vi "ToRepo.vi"(8 "error in":errorcluster, 9 "to repo cluster":T1, 10 "repository in":refnum<class "NISE_CEF_Repository.lvclass">, 11 "node in":refnum<class "Pages.lvclass">) -> (0 "error out":errorcluster, 2 "repository out":refnum<class "NISE_CEF_Repository.lvclass">, 3 "node out":refnum<class "Pages.lvclass">)   [LabVIEW 2015, in "Pages.lvclass"]
doc: "Transfers the information from the tree node into the repo. How it is stored in the repo depends on the Repo.Copyright 2015 National Instruments Corporation\n\nLicensed under the Apache License, Version 2.0 (the \"License\"); you may not use this file except in compliance with the License. You may obtain a copy of the License at http://www.apache.org/licenses/LICENSE-2.0\nUnless required by applicable law or agreed to in writing, software distributed under the License is distributed on an \"AS IS\" BASIS, WITHOUT WARRANTIES OR CONDITIONS OF ANY KIND, either express or implied. See the License for the specific language governing permissions and limitations under the License."
uses:
  Pages.lvclass
  <vilib>/NI/Configuration Framework/Repository/NISE_CEF_Repository.lvclass
  <vilib>/NI/Configuration Framework/Node/ToRepoCluster.ctl
  CustomDeviceRepo/CustomDeviceRepo.lvclass
  <vilib>/NI/Configuration Framework/Node/NISE_CEF_Node.lvclass/NISE_CEF_Node.ctl
  Page/Page.lvclass
  Custom Device Type Defs/Page Properties.ctl
  XML Controls/Path Cluster.ctl
  XML Controls/help.ctl
  Custom Device Type Defs/ActionVIs Properties.ctl
  Custom Device Type Defs/ButtonLists Properties.ctl
  XML Controls/Button Type.ctl
  XML Controls/Dependency three item small.ctl
  Custom Device Type Defs/RunTimeMenus Properties.ctl
  XML Controls/Execution Types.ctl
  Page/Page.lvclass/Page.ctl
  RunTimeObjects/RunTimeObjectsSection.lvclass
  RunTimeObjects/RunTimeObjectsSection.lvclass/RunTimeObjectsSection.ctl
  ActionVI/ActionVI.lvclass
  ActionVI/ActionVI.lvclass/ActionVI.ctl
  RunTimeButton/RunTimeButton.lvclass
  RunTimeButton/RunTimeButton.lvclass/RunTimeButton.ctl
  RunTimeMenuItem/RunTimeMenuItem.lvclass
  RunTimeMenuItem/RunTimeMenuItem.lvclass/RunTimeMenuItem.ctl
  CustomDeviceRepo/CustomDeviceRepo.lvclass/CustomDeviceRepo.ctl
  ActionVI/Read ActionVIType.vi
  ActionVI/Read Action VI Properties.vi
  RunTimeButton/Read Button Properties.vi
  RunTimeMenuItem/Read Run Time Menu Properties.vi
  RunTimeObjects/Read RunTimeObjectType.vi
  <vilib>/NI/Configuration Framework/Node/ReadChildren.vi
  Page/Read General Page Properties.vi
  CustomDeviceRepo/Write All Pages Properties.vi
  <vilib>/NI/Configuration Framework/Node/NISE_CEF_Node.lvclass
  Configuration Tool.lvlib
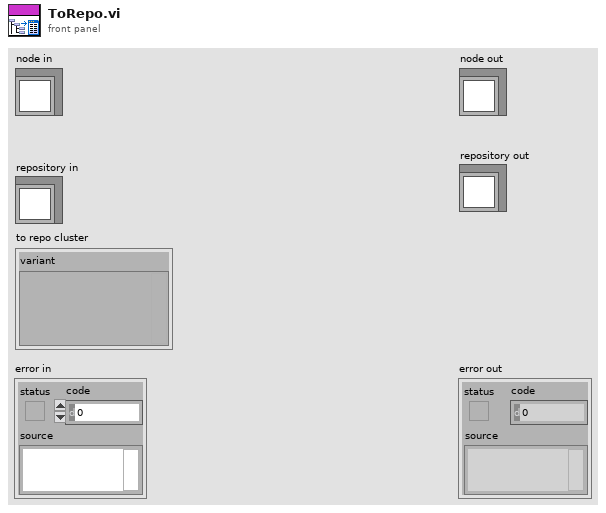
[diagram p1: front panel]
types:
  T1 = typedef "NISE_CEF_Node.lvclass/ToRepoCluster.ctl" = cluster{"variant":variant}
  T2 = typedef "NISE_CEF_Node.lvclass/NodeRef.ctl" = refnum<data-value>
  T3 = typedef "Page Properties.ctl" = cluster{"Name":string, "Disallow Renaming":bool, "Delete Protection":bool, "Exlcude from Alphabetical order":bool, "Allow Multi-Selection":bool, "GUID":string, "Parent GUIDs":string[], "Glyph":T4, "Inactive Glyph":T4, "Broken Glyph":T4, "Item to Launch":T4, "Additional Information":string, "Copy":enum16{"copy", "disabled"}, "Paste":enum16{"Create", "CreatIfNotExists_GUID", "CreatIfNotExists_Name", "Replace", "Dialog"}, "Help":T5}
  T4 = typedef "Configuration Tool.lvlib/Path Cluster.ctl" = cluster{"Path":path, "Path Type":enum16{"Absolute", "To Base", "To Common Doc Dir", "To Application Data Dir"}}
  T5 = typedef "Configuration Tool.lvlib/help.ctl" = cluster{"Item to Launch":T4, "Section":string, "File Type":enum16{"chm", "other"}}
  T6 = typedef "ActionVIs Properties.ctl" = cluster{"Action VI On Delete":T4, "Action VI On Load":T4, "Action VI On Paste":T4, "Action VI On Target Type Change":T4, "Action VI On Delete Request":T4, "Action VI On Compile":T4, "Action VI On System Shutdown":T4, "Action VI On Save":T4, "Action VI On Download":T4}
  T7 = typedef "ButtonLists Properties.ctl" = cluster{"ID":string, "Glyph":T4, "Button Type":T8, "Referenced GUID":string, "Button Text":string, "Caption":string, "Tip Strip":string, "Documentation":string, "Dependency":T9}
  T8 = typedef "Configuration Tool.lvlib/Button Type.ctl" = enum16{"Action", "Dialog", "Page", "Notification", "Separator"}
  T9 = typedef "Configuration Tool.lvlib/Dependency three item small.ctl" = cluster{"File Path Control":path, "Path Type":enum16{"Absolute", "To Base", "To Common Doc Dir", "To Application Data Dir"}, "Behavior":enum16{"Static", "Dynamic"}}
  T10 = typedef "RunTimeMenus Properties.ctl" = cluster{"GUID":string, "Execution":T11, "MinNrOfChilds":u32, "Name":string, "Item to Launch":T4, "Dependency":T9, "Custom Population":T4, "Menu Item Type":enum16{"Action", "VI", "Separator", "Custom"}, "Behavior":enum16{"Nothing", "Open Front Panel"}, "Position":enum16{"Centered", "Mouse Pointer"}}
  T11 = typedef "Configuration Tool.lvlib/Execution Types.ctl" = enum16{"silent", "modal", "floating", "default"}
  T12 = cluster{"General Page Properties":T3, "ActionVIs Properties":T6, "Button List Properties":T7[], "RunTime Menus Properties":T10[]}
  T13 = typedef "RunTimeObjectTypes.ctl" = enum16{"ActionVIs", "ButtonList", "RunTimeMenu"}
  T14 = typedef "ActionVITypes.ctl" = enum16{"OnDelete", "OnLoad", "OnSystemShutdown", "OnSave", "OnDownload", "OnPaste", "OnTargetTypeChange", "OnDeleteRequest", "OnCompile"}
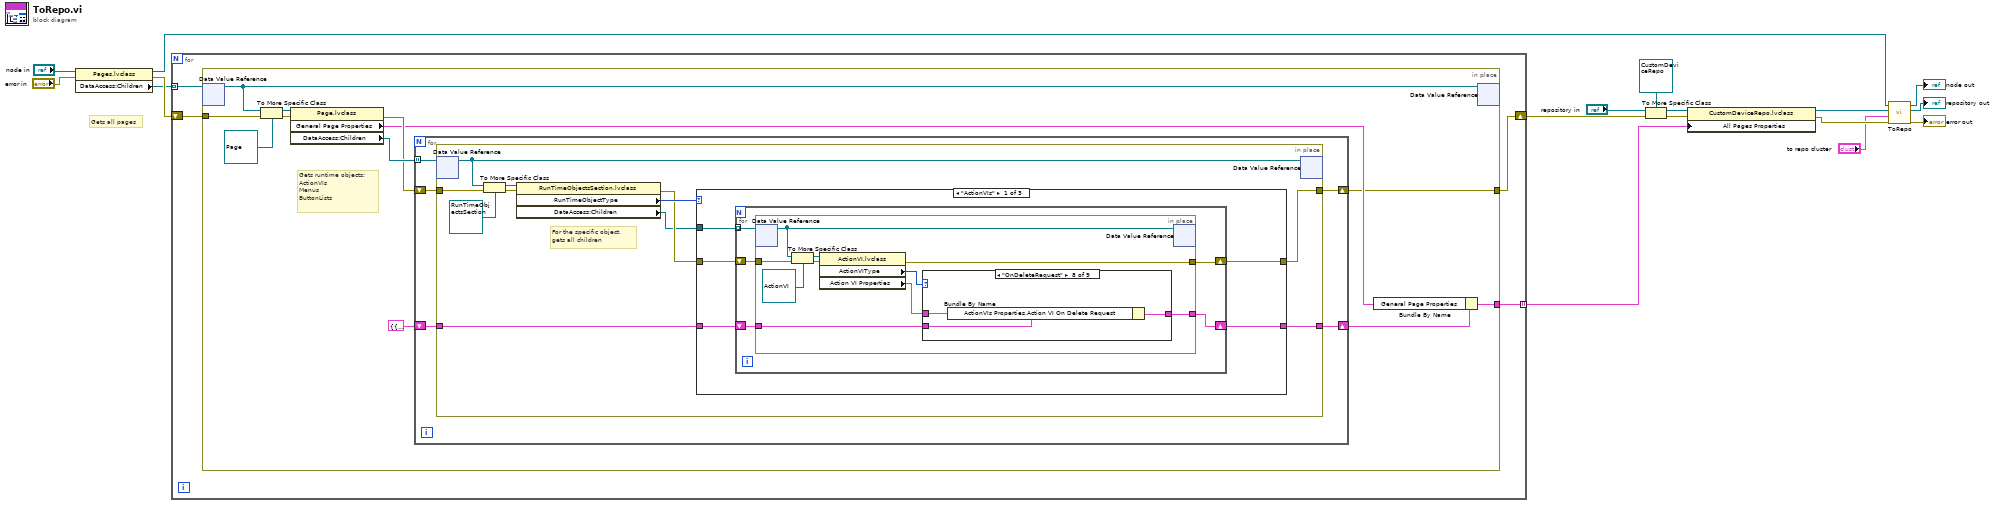
[diagram p0: block diagram]
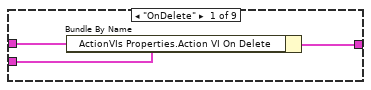
[diagram p2: hidden frame]
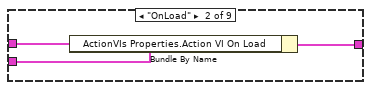
[diagram p3: hidden frame]
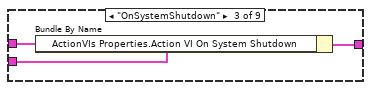
[diagram p4: hidden frame]
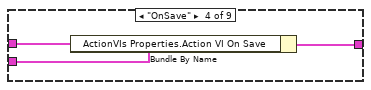
[diagram p5: hidden frame]
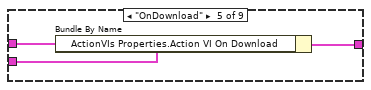
[diagram p6: hidden frame]
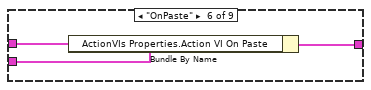
[diagram p7: hidden frame]
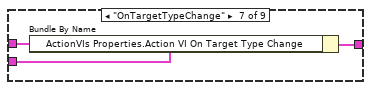
[diagram p8: hidden frame]
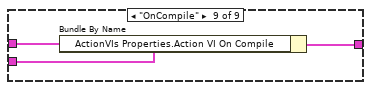
[diagram p9: hidden frame]
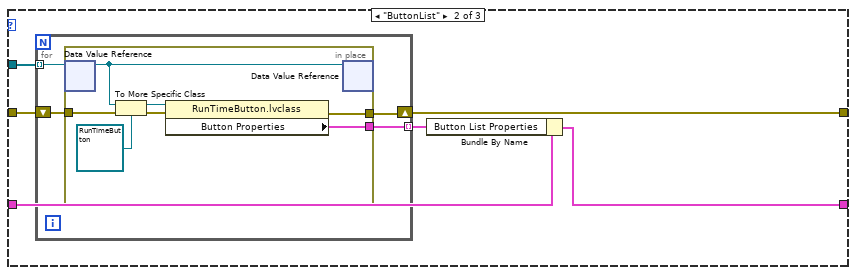
[diagram p10: hidden frame]
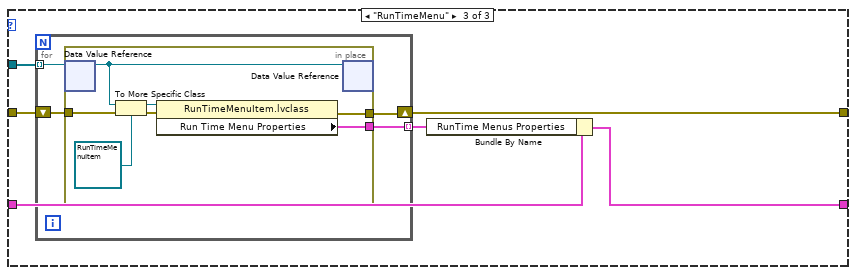
[diagram p11: hidden frame]
diagram:
  # "Gets all pages"
  n1 = property class="Pages.lvclass"(reference="node in", error in="error in") -> (reference out=w6:refnum<class "Pages.lvclass">, error out=w12:errorcluster, "DataAccess:Children"=w11:T2[])
  n2 = for {
    shift-right: [w18] -> w10
    shift-left: w12 -> [w20]
    tunnel: w11 -> [w21] mode=indexing
    tunnel: [w19] -> w1 mode=indexing
    n3 = in-place {
      in-place-border: w20 -> [w33]
      in-place-border: [w23] -> w19
      in-place-border: [w22] -> w18
      # "Gets runtime objects:\nActionVIs\nMenus\nButtonLists"
      n4 = in-place-dvr #1(w21) -> (w32:refnum<class "NISE_CEF_Node.lvclass">)  [unwired: 1 out]
      n5 = To More Specific Class(target class=refnum<class "Page.lvclass"> refnum ("Page.lvclass"), reference=w32, error in=w33) -> (specific class reference=w31:refnum<class "Page.lvclass">, error out=w30:errorcluster)
      n6 = property class="Page.lvclass"(reference=w31, error in=w30) -> (error out=w27:errorcluster, "General Page Properties"=w24:T3, "DataAccess:Children"=w28:T2[])  [unwired: 1 out]
      n7 = for {
        tunnel: w28 -> [w38] mode=indexing
        shift-right: [w35] -> w22
        shift-left: w27 -> [w37]
        shift-right: [w34] -> w25
        shift-left: T12 {"General Page Properties"={"Name"="", "Disallow Renaming"=FALSE, "Delete Protection"=FALSE, "Exlcude from Alphabetical order"=FALSE, "Allow Multi-Selection"=FALSE, "GUID"="", "Parent GUIDs"=[], "Glyph"={"Path"=path "", "Path Type"=enum."Absolute"}, "Inactive Glyph"={"Path"=path "", "Path Type"=enum."Absolute"}, "Broken Glyph"={"Path"=path "", "Path Type"=enum."Absolute"}, "Item to Launch"={"Path"=path "", "Path Type"=enum."Absolute"}, "Additional Information"="", "Copy"=enum."copy", "Paste"=enum."Create", "Help"={"Item to Launch"={"Path"=path "", "Path Type"=enum."Absolute"}, "Section"="", "File Type"=enum."chm"}}, "ActionVIs Properties"={"Action VI On Delete"={"Path"=path "", "Path Type"=enum."Absolute"}, "Action VI On Load"={"Path"=path "", "Path Type"=enum."Absolute"}, "Action VI On Paste"={"Path"=path "", "Path Type"=enum."Absolute"}, "Action VI On Target Type Change"={"Path"=path "", "Path Type"=enum."Absolute"}, "Action VI On Delete Request"={"Path"=path "", "Path Type"=enum."Absolute"}, "Action VI On Compile"={"Path"=path "", "Path Type"=enum."Absolute"}, "Action VI On System Shutdown"={"Path"=path "", "Path Type"=enum."Absolute"}, "Action VI On Save"={"Path"=path "", "Path Type"=enum."Absolute"}, "Action VI On Download"={"Path"=path "", "Path Type"=enum."Absolute"}}, "Button List Properties"=[], "RunTime Menus Properties"=[]} ("Page Properties") -> [w36]
        n8 = in-place {
          in-place-border: w37 -> [w49]
          in-place-border: w36 -> [w41]
          in-place-border: [w40] -> w35
          in-place-border: [w39] -> w34
          # "For the specific object,\ngets all children"
          n9 = in-place-dvr #2(w38) -> (w48:refnum<class "NISE_CEF_Node.lvclass">)  [unwired: 1 out]
          n10 = To More Specific Class(target class=refnum<class "RunTimeObjectsSection.lvclass"> refnum ("RunTimeObjectsSection.lvclass"), reference=w48, error in=w49) -> (specific class reference=w47:refnum<class "RunTimeObjectsSection.lvclass">, error out=w46:errorcluster)
          n11 = property class="RunTimeObjectsSection.lvclass"(reference=w47, error in=w46) -> (error out=w43:errorcluster, "RunTimeObjectType"=w44:T13, "DataAccess:Children"=w42:T2[])  [unwired: 1 out]
          n12 = case shown="\"ActionVIs\"" w44 {
            tunnel: [w51 w102 w114] -> w40
            tunnel: w41 -> [w52 w101 w117]
            tunnel: [w50 w99 w115] -> w39
            tunnel: w43 -> [w53 w98 w118]
            tunnel: w42 -> [w54 w97 w119]
            frame "ActionVIs" {
              n13 = for {
                shift-right: [w58] -> w51
                shift-left: w53 -> [w59]
                tunnel: w54 -> [w57] mode=indexing
                shift-right: [w55] -> w50
                shift-left: w52 -> [w56]
                n14 = in-place {
                  in-place-border: w59 -> [w69]
                  in-place-border: [w65] -> w58
                  in-place-border: w56 -> [w63]
                  in-place-border: [w62] -> w55
                  n15 = in-place-dvr #3(w57) -> (w68:refnum<class "NISE_CEF_Node.lvclass">)  [unwired: 1 out]
                  n16 = To More Specific Class(target class=refnum<class "ActionVI.lvclass"> refnum ("ActionVI.lvclass"), reference=w68, error in=w69) -> (specific class reference=w67:refnum<class "ActionVI.lvclass">, error out=w66:errorcluster)
                  n17 = property class="ActionVI.lvclass"(reference=w67, error in=w66) -> (error out=w65:errorcluster, "ActionVIType"=w61:T14, "Action VI Properties"=w60:T4)  [unwired: 1 out]
                  n18 = case shown="\"OnDeleteRequest\"" w61 {
                    tunnel: w63 -> [w72 w75 w78 w81 w84 w87 w90 w93 w96]
                    tunnel: [w71 w74 w77 w80 w83 w86 w89 w92 w95] -> w62
                    tunnel: w60 -> [w70 w73 w76 w79 w82 w85 w88 w91 w94]
                    frame "OnDelete" {
                      n19 = Bundle By Name(cluster=w72, "ActionVIs Properties.Action VI On Delete"=w70) -> (w71:T12)
                    }
                    frame "OnLoad" {
                      n20 = Bundle By Name(cluster=w75, "ActionVIs Properties.Action VI On Load"=w73) -> (w74:T12)
                    }
                    frame "OnSystemShutdown" {
                      n21 = Bundle By Name(cluster=w78, "ActionVIs Properties.Action VI On System Shutdown"=w76) -> (w77:T12)
                    }
                    frame "OnSave" {
                      n22 = Bundle By Name(cluster=w81, "ActionVIs Properties.Action VI On Save"=w79) -> (w80:T12)
                    }
                    frame "OnDownload" {
                      n23 = Bundle By Name(cluster=w84, "ActionVIs Properties.Action VI On Download"=w82) -> (w83:T12)
                    }
                    frame "OnPaste" {
                      n24 = Bundle By Name(cluster=w87, "ActionVIs Properties.Action VI On Paste"=w85) -> (w86:T12)
                    }
                    frame "OnTargetTypeChange" {
                      n25 = Bundle By Name(cluster=w90, "ActionVIs Properties.Action VI On Target Type Change"=w88) -> (w89:T12)
                    }
                    frame "OnDeleteRequest" {
                      n26 = Bundle By Name(cluster=w93, "ActionVIs Properties.Action VI On Delete Request"=w91) -> (w92:T12)
                    }
                    frame "OnCompile" {
                      n27 = Bundle By Name(cluster=w96, "ActionVIs Properties.Action VI On Compile"=w94) -> (w95:T12)
                    }
                  }
                  n28 = in-place-dvr #3(w68) -> ()  [unwired: 2 out]
                }
              }
            }
            frame "ButtonList" {
              n29 = for {
                shift-right: [w104] -> w102
                shift-left: w98 -> [w106]
                tunnel: [w105] -> w100 mode=indexing
                tunnel: w97 -> [w103] mode=indexing
                n30 = in-place {
                  in-place-border: w106 -> [w113]
                  in-place-border: [w108] -> w105
                  in-place-border: [w107] -> w104
                  n31 = in-place-dvr #4(w103) -> (w112:refnum<class "NISE_CEF_Node.lvclass">)  [unwired: 1 out]
                  n32 = To More Specific Class(target class=refnum<class "RunTimeButton.lvclass"> refnum ("RunTimeButton.lvclass"), reference=w112, error in=w113) -> (specific class reference=w110:refnum<class "RunTimeButton.lvclass">, error out=w109:errorcluster)
                  n33 = property class="RunTimeButton.lvclass"(reference=w110, error in=w109) -> (error out=w107:errorcluster, "Button Properties"=w108:T7)  [unwired: 1 out]
                  n34 = in-place-dvr #4(w112) -> ()  [unwired: 2 out]
                }
              }
              n35 = Bundle By Name(cluster=w101, "Button List Properties"=w100) -> (w99:T12)
            }
            frame "RunTimeMenu" {
              n36 = for {
                shift-right: [w121] -> w114
                shift-left: w118 -> [w123]
                tunnel: [w122] -> w116 mode=indexing
                tunnel: w119 -> [w120] mode=indexing
                n37 = in-place {
                  in-place-border: w123 -> [w130]
                  in-place-border: [w126] -> w122
                  in-place-border: [w125] -> w121
                  n38 = in-place-dvr #5(w120) -> (w129:refnum<class "NISE_CEF_Node.lvclass">)  [unwired: 1 out]
                  n39 = To More Specific Class(target class=refnum<class "RunTimeMenuItem.lvclass"> refnum ("RunTimeMenuItem.lvclass"), reference=w129, error in=w130) -> (specific class reference=w128:refnum<class "RunTimeMenuItem.lvclass">, error out=w127:errorcluster)
                  n40 = property class="RunTimeMenuItem.lvclass"(reference=w128, error in=w127) -> (error out=w125:errorcluster, "Run Time Menu Properties"=w126:T10)  [unwired: 1 out]
                  n41 = in-place-dvr #5(w129) -> ()  [unwired: 2 out]
                }
              }
              n42 = Bundle By Name(cluster=w117, "RunTime Menus Properties"=w116) -> (w115:T12)
            }
          }
          n43 = in-place-dvr #2(w48) -> ()  [unwired: 2 out]
        }
      }
      n44 = Bundle By Name(cluster=w25, "General Page Properties"=w24) -> (w23:T12)
      n45 = in-place-dvr #1(w32) -> ()  [unwired: 2 out]
    }
  }
  n46 = To More Specific Class(target class=refnum<class "CustomDeviceRepo.lvclass"> refnum ("CustomDeviceRepo.lvclass"), reference="repository in", error in=w10) -> (specific class reference=w15:refnum<class "CustomDeviceRepo.lvclass">, error out=w14:errorcluster)
  n47 = property class="CustomDeviceRepo.lvclass"(reference=w15, error in=w14, "All Pages Properties"=w1) -> (reference out=w5:refnum<class "CustomDeviceRepo.lvclass">, error out=w4:errorcluster)
  n48 = call-parent "ToRepo.vi"("error in"=w4, "to repo cluster"="to repo cluster", "repository in"=w5, "node in"=w6) -> ("error out"=→"error out":errorcluster, "repository out"=→"repository out":refnum<class "NISE_CEF_Repository.lvclass">, "node out"=→"node out":refnum<class "Pages.lvclass">)  [unwired: 5 in]
